vi "delay_sleep_deprivation_start_by_x_images.vi"(0 "Input \nParameters":T4={"Frame rate (ms)"=2000, "Worm strain"="N2", "# Images"=0, "State"=enum."Image acquisition", "Time elapsed"=0.0, "Max_num_runs"=100000, "#TTL"=0, "Time of start TTL"=100000, "ImSub Value"=0, "Time of last TTL"=0, "Number of Columns"=2, "Number of Rows"=2, "# AdjacentTTL"=0, "Sleep deprivation status"="", "Sleep Detection"=FALSE, "# Sleep detections"=0, "Time of first sleep detection"=0, "Time max # adjacent TTL"=0, "Image t-1"=[], "Image t"=[]} {"Number of Rows" items=["1"=1, "2"=2, "3"=3, "4"=4]; "Number of Columns" items=["1"=1, "2"=2, "3"=3, "4"=4]}, 3 "Deprivation\nparameters":T1={"Frame Row"=0, "Kstd"=40.0, "# Images for\nsleep detection"=10, "Kmean"=1.5, "Start time of sleep detection (images):"=1000, 0, "Length (images)"=3600, "# TTL"=10000, "Delay by x images after first detection"=0, "Between TTL pulses"=0, "\nby x detections"=9, "# Total immobility\n detections"=0, "max # adjacent\nTTL"=0.0, "TTL x start\ntime deprivation\n"=0.0, "Max #\nadjacent TTL"=10000, " Ca2+\nmode"=0} {"?" items=["1", "2", "3", "4"]; "Frame Row" items=["1", "2", "3", "4"]}) -> (5 "Output \nParameters":T3={"Frame rate (ms)"=2000, "Worm strain"="N2", "Time t"=0, "State"=enum."Image acquisition", "Time elapsed"=0.0, "Max_num_runs"=100000, "#TTL"=0, "Time of start TTL"=100000, "ImSub Value"=0, "Time of last TTL"=0, "Number of Columns"=2, "Number of Rows"=2, "# AdjacentTTL"=0, "Sleep deprivation status"="", "Sleep Detection"=FALSE, "# Sleep detections"=0, "Time of first sleep detection"=0, "Time max # adjacent TTL"=0, "Image t-1"=[], "Image t"=[]} {"Number of Rows" items=["1"=1, "2"=2, "3"=3, "4"=4]; "Number of Columns" items=["1"=1, "2"=2, "3"=3, "4"=4]})   [LabVIEW 2011]
uses:
  state.ctl
panel:
  # "Sleep deprivation settings"
  # "Select deprivation animal"
  # "Row"
  # "Column"
  # "Sleep detection parameters"
  # "Sleep deprivation parameters"
  # "Delay deprivation start:"
  # "Pause deprivation (images):"
  # "Stop deprivation after:"
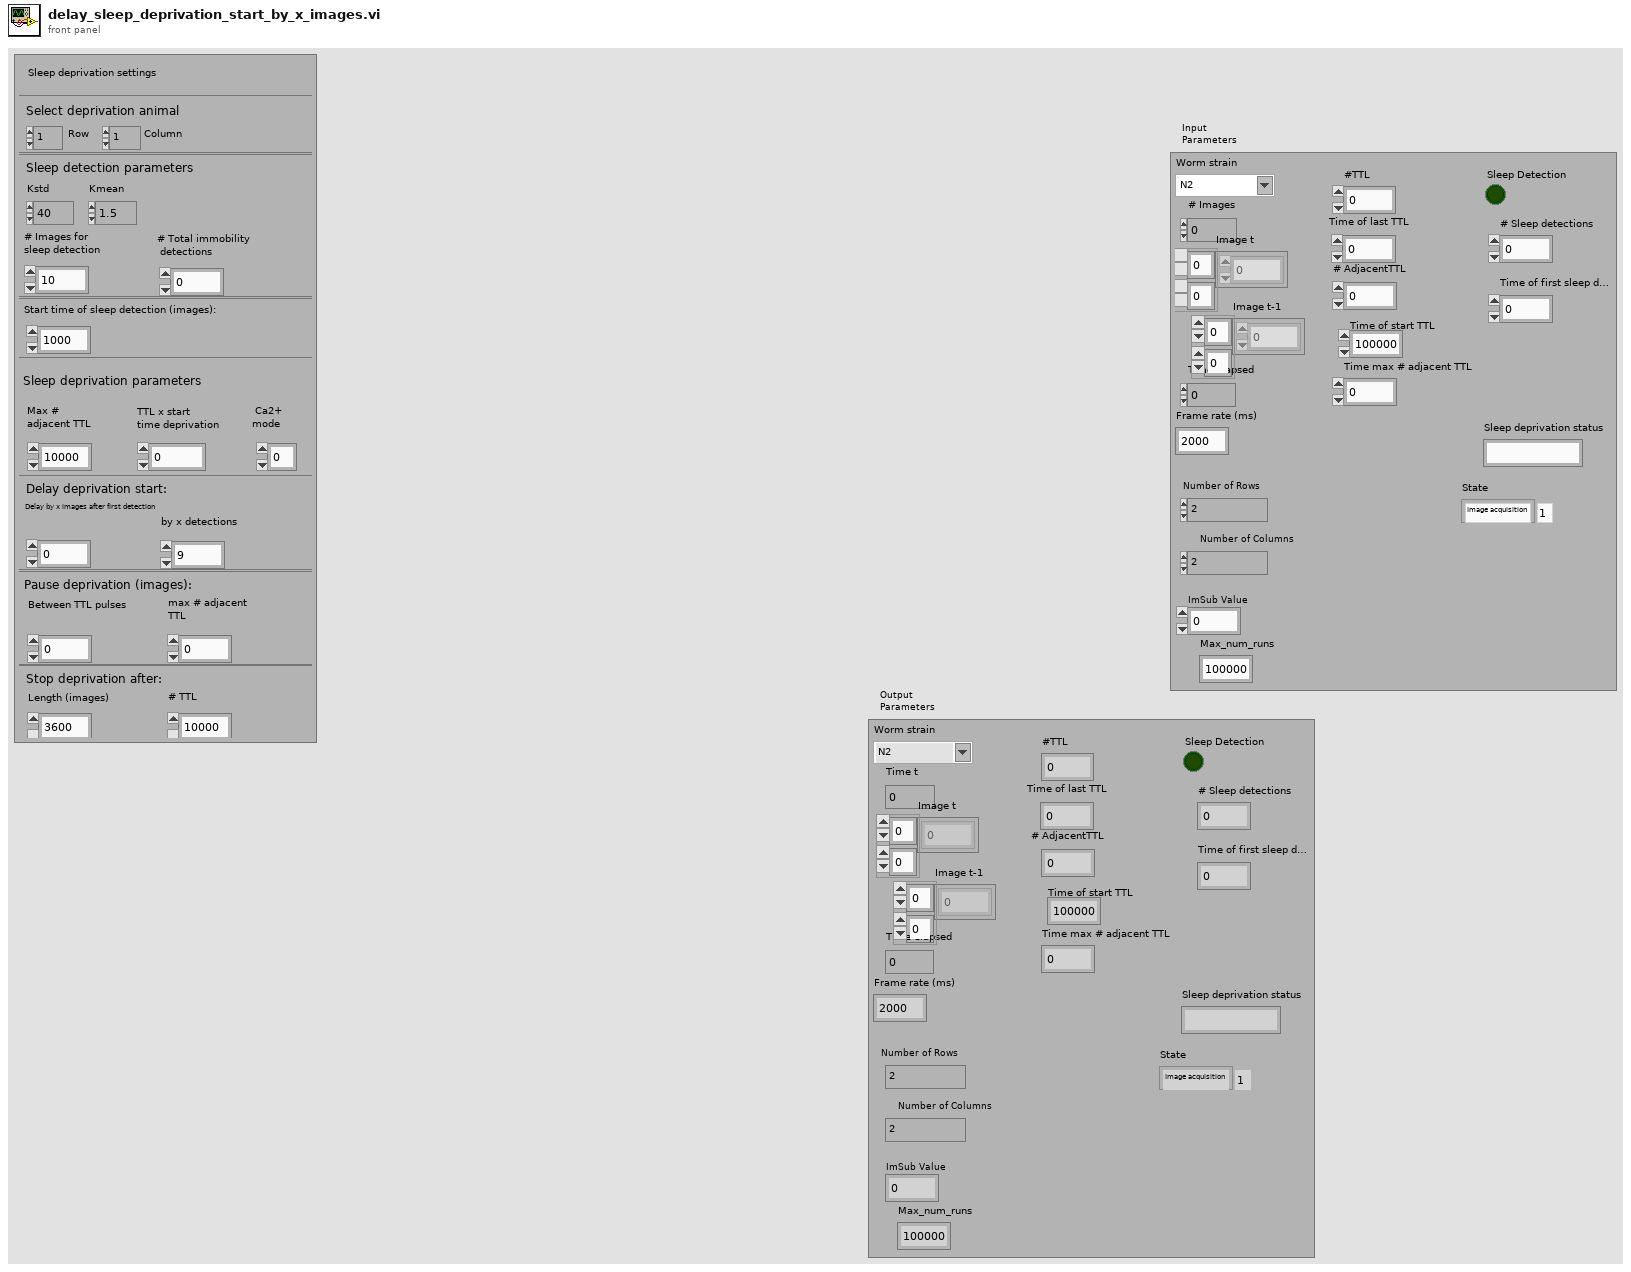
[diagram p1: front panel]
types:
  T1 = cluster{"Frame Row":u32, "Kstd":dbl, "# Images for\nsleep detection":i32, "Kmean":dbl, "Start time of sleep detection (images):":i32, u32, "Length (images)":i32, "# TTL":i32, "Delay by x images after first detection":i32, "Between TTL pulses":i32, "\nby x detections":i32, "# Total immobility\n detections":i32, "max # adjacent\nTTL":dbl, "TTL x start\ntime deprivation\n":dbl, "Max #\nadjacent TTL":i32, " Ca2+\nmode":i32}
  T2 = typedef "state.ctl" = enum16{"Initialize measurement", "Image acquisition", "Image processing", "Sleep detection", "Control TTL protocol ", "Sleep deprivation", "Update image & exit condition", "Wait "}
  T3 = cluster{"Frame rate (ms)":u32, "Worm strain":string, "Time t":i32, "State":T2, "Time elapsed":dbl, "Max_num_runs":i32, "#TTL":i32, "Time of start TTL":i32, "ImSub Value":i32, "Time of last TTL":i32, "Number of Columns":u32, "Number of Rows":u32, "# AdjacentTTL":i32, "Sleep deprivation status":string, "Sleep Detection":bool, "# Sleep detections":i32, "Time of first sleep detection":i32, "Time max # adjacent TTL":i32, "Image t-1":i32[][], "Image t":i32[][]}
  T4 = cluster{"Frame rate (ms)":u32, "Worm strain":string, "# Images":i32, "State":T2, "Time elapsed":dbl, "Max_num_runs":i32, "#TTL":i32, "Time of start TTL":i32, "ImSub Value":i32, "Time of last TTL":i32, "Number of Columns":u32, "Number of Rows":u32, "# AdjacentTTL":i32, "Sleep deprivation status":string, "Sleep Detection":bool, "# Sleep detections":i32, "Time of first sleep detection":i32, "Time max # adjacent TTL":i32, "Image t-1":i32[][], "Image t":i32[][]}
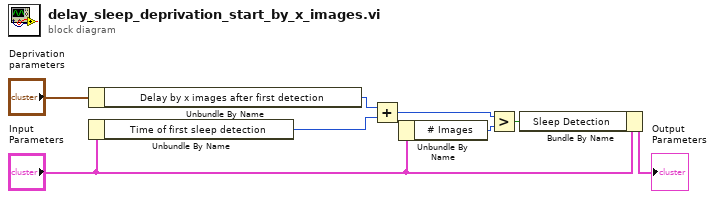
[diagram p0: block diagram]
diagram:
  n1 = Unbundle By Name("Deprivation\nparameters") -> ("Delay by x images after first detection"=w8:i32)
  n2 = Unbundle By Name("Input \nParameters") -> ("Time of first sleep detection"=w7:i32)
  n3 = Add(x=w8, y=w7) -> (x+y=w5:i32)
  n4 = Unbundle By Name("Input \nParameters") -> ("# Images"=w6:i32)
  n5 = Greater?(x=w5, y=w6) -> (0:w4:bool)
  n6 = Bundle By Name(cluster="Input \nParameters", "Sleep Detection"=w4) -> (→"Output \nParameters":T4)
